vi "CRYRename Data by Step Rename.vi"(11 "Tree VI No.":i32) -> ()   [LabVIEW 2013]
uses:
  CRYCurveLibrary/Global/CRYCurve Library Global.vi
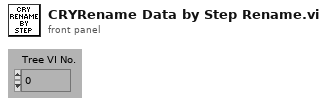
[diagram p1: front panel]
types:
  T1 = typedef "CRYStep.ctl" = cluster{"No.VI":i32, "Category":string, "StepName":string, "Seq setup flattened":string, "Comment":string, "Steps config.":bool[], "Jump config":i32[], "Start":dbl, "Increment":dbl, "Name":string, "Unit":string, "Y data":u16, "Y prefix":string, "Y dB ref":dbl, "Y unit":string, "Repeat State Array":cluster{"Start":dbl, "Increment":dbl, "Count":i32, "Num":i32}[]}
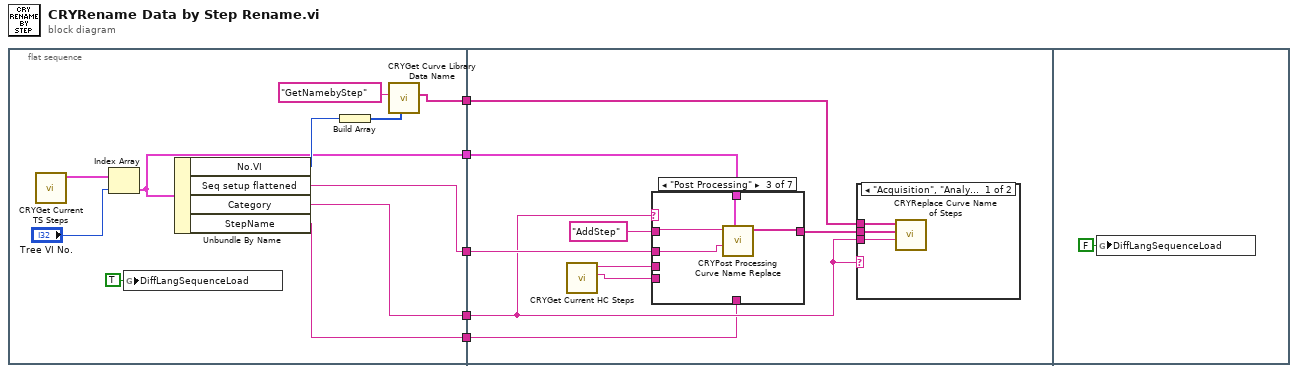
[diagram p0: block diagram]
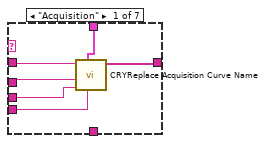
[diagram p3: hidden frame]
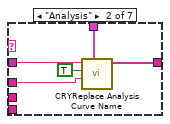
[diagram p4: hidden frame]
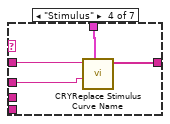
[diagram p5: hidden frame]
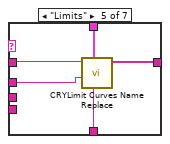
[diagram p6: hidden frame]
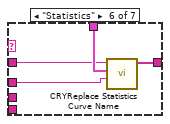
[diagram p7: hidden frame]
diagram:
  n1 = flat-sequence {
    tunnel: [w8] -> w5
    tunnel: [w9] -> w4
    tunnel: [w10] -> w3
    tunnel: [w11] -> w2
    tunnel: [w12] -> w1
    tunnel: w5 -> [w25]
    tunnel: w4 -> [w21]
    tunnel: w3 -> [w18]
    tunnel: w2 -> [w17]
    tunnel: w1 -> [w23]
    frame #0 {
      n2 = call "CRYGet Current TS Steps.vi"() -> ("Steps"=w15:T1[])  [unwired: 1 in, 10 out]
      n3 = Index Array(array=w15, index="Tree VI No.") -> (element=w12:T1)
      n4 = global write "CRYCurve Library Global.vi" "DiffLangSequenceLoad"(TRUE ("DiffLangSequenceLoad")) -> ()
      n5 = Unbundle By Name(w12) -> ("No.VI"=w16:i32, "Seq setup flattened"=w9:string, "Category"=w10:string, "StepName"=w11:string)
      n6 = Build Array(w16) -> (w13:i32[])
      n7 = call "CRYGet Curve Library Data Name.vi"("nData"=w13, "sAction"="GetNamebyStep" ("sOption")) -> ("sNames"=w8:string[])  [unwired: 6 in, 3 out]
    }
    frame #1 {
      n8 = call "CRYGet Current HC Steps.vi"() -> ("Calibration setup flattened Out"=w19:string, "Hardware setup flattened Out"=w20:string)  [unwired: 10 in]
      n9 = case shown="\"Post Processing\"" w18 {
        tunnel: "AddStep" ("Type In") -> [w33 w38 w41 w47 w50 w54 _]
        tunnel: w23 -> [w34 w37 w43 w46 w52 w56 _]
        tunnel: [w29 w36 w42 w45 w51 w55 _] -> w22
        tunnel: w21 -> [w32 w35 w40 w44 w49 w53 _]
        tunnel: w20 -> [w31 _ _ _ _ _ _]
        tunnel: w19 -> [w30 _ _ _ _ _ _]
        tunnel: w17 -> [_ _ _ _ w48 _ _]
        frame "Acquisition" {
          n10 = call "CRYReplace Acquisition Curve Name.vi"("Calibration in"=w30, "Setup in"=w34, "Hardware Setup In"=w31, "Step Setup In"=w32, "Type In"=w33) -> ("Inserted Names Out"=w29:string[])  [unwired: 4 in, 2 out]
        }
        frame "Analysis" {
          n11 = call "CRYReplace Analysis Curve Name.vi"("Setup in"=w37, "Step Setup In"=w35, "InsertSocket?"=TRUE, "Type In"=w38) -> ("Inserted Names Out"=w36:string[])  [unwired: 3 in, 4 out]
        }
        frame "Post Processing" {
          n12 = call "CRYPost Processing Curve Name Replace.vi"("Setup in"=w43, "Step Setup in"=w40, "Type In"=w41) -> ("Inserted Names Out"=w42:string[])  [unwired: 8 in]
        }
        frame "Stimulus" {
          n13 = call "CRYReplace Stimulus Curve Name.vi"("Setup in"=w46, "Step Setup In"=w44, "Type In"=w47) -> ("Inserted Names Out"=w45:string[])  [unwired: 8 in]
        }
        frame "Limits" {
          n14 = call "CRYLimit Curves Name Replace.vi"("StepName"=w48, "Setup in"=w52, "Step Set up In"=w49, "Type In"=w50) -> ("Inserted Names Out"=w51:string[])  [unwired: 7 in]
        }
        frame "Statistics" {
          n15 = call "CRYReplace Statistics Curve Name.vi"("Step Set up In"=w53, "Setup in"=w56, "Type In"=w54) -> ("Inserted Names Out"=w55:string[])  [unwired: 7 in, 1 out]
        }
        frame Default {
        }
      }
      n16 = case shown="\"Acquisition\", \"Analysis\", \"Limits\", \"Post Processing\", \"Statistics\", \"Stimulus\"" w18 {
        tunnel: w25 -> [w28 _]
        tunnel: w18 -> [w27 _]
        tunnel: w22 -> [w26 _]
        frame "Acquisition", "Analysis", "Limits", "Post Processing", "Statistics", "Stimulus" {
          n17 = call "CRYReplace Curve Name of Steps.vi"("Step Category"=w27, "New Name"=w26, "Old Name"=w28) -> ()  [unwired: 8 in, 1 out]
        }
        frame Default {
        }
      }
    }
    frame #2 {
      n18 = global write "CRYCurve Library Global.vi" "DiffLangSequenceLoad"(FALSE ("DiffLangSequenceLoad")) -> ()
    }
  }
